vi "FaulhaberV3AsciiCommunication.vi"(8 "error in (no error)":errorcluster, 10 "Befehl":string="Statusword?", 11 "VISA resource name":refnum<visa-resource-name>="COM10") -> (0 "error out":errorcluster={"status"=FALSE, "code"=1073676293, "source"="VISA Read in FaulhaberCommunication.vi->Faulhaber_Standalone.vi"}, 1 "returnValue":i32 format="%.0x", 2 "return":string="5000\r\n", 3 "VISA resource name out":refnum<visa-resource-name>="COM10")   [LabVIEW 2011]
uses:
  FaulaberType.ctl
panel:
  out "type":T1=enum."R"
  in  "Knoten":u8=1
  out "Befehl 2":T2(ring)
  out "Value":i32 format="%.0x"
  out "Index":u32 format="%04x"
  # "2025 new binary interface"
  # "Modes of operation=1\nControlword=0xF\nControlword?\nStatusword?\nTarget position=12345\nControlword=0xF\nControlword=0xF\nPosition actual value?"
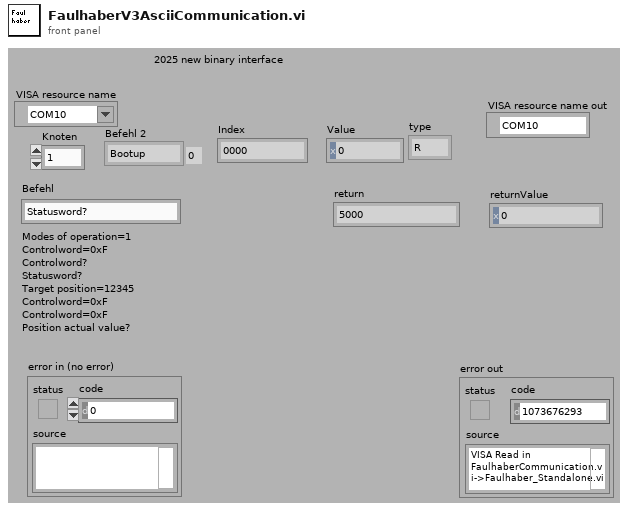
[diagram p1: front panel]
types:
  T1 = typedef "FaulaberType.ctl" = enum8{"unknown", "none", "S8", "S16", "S32", "U8", "U16", "U32", "R", "string"}
  T2 = enum8{"Bootup", "SDORead", "SDOWrite", "SDOErrror", "Controlword", "Statusword", "TraceLog", "Emcy", "SDOBlockReadInit", "SDOBlockReadUpload", "SDOBlockReadEnd", "SDOBlockWriteInit", "SDOBlockWriteDownload", "SDOBlockWriteEnd"}
  T3 = typedef "FaulhaberAccess.ctl" = enum16{"unknown", "ro", "rw", "wo", "const"}
  T4 = cluster{"ID":u32, "Name":string, "type":T1, "rw":T3, "lowLimit":string, "highLimit":string, "Default":string, "Kommentart":string}[]
  T5 = cluster{"ID":u32, "Name":string, "type":T1, "rw":T3, "lowLimit":string, "highLimit":string, "Default":string, "Kommentart":string}
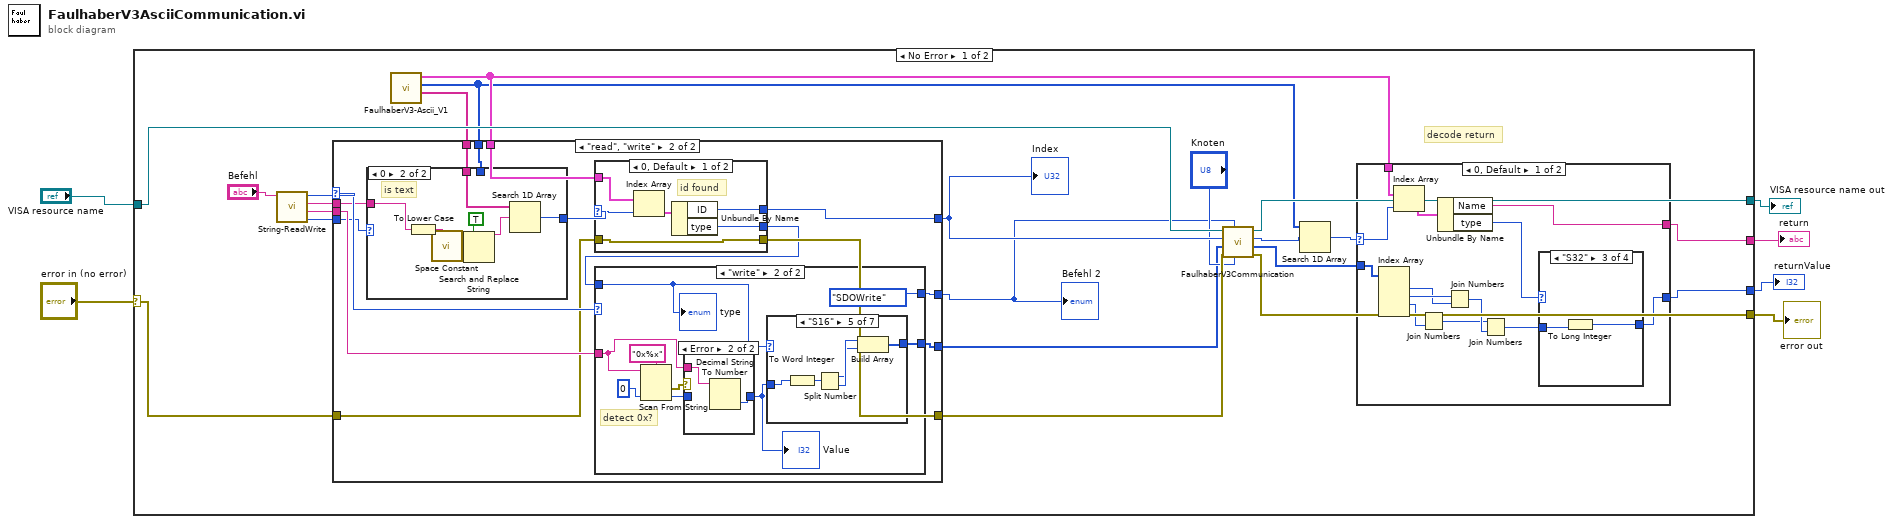
[diagram p0: block diagram]
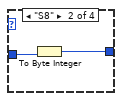
[diagram p3: hidden frame]
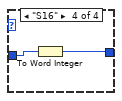
[diagram p4: hidden frame]
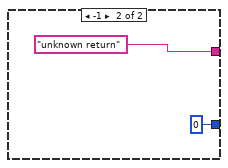
[diagram p5: hidden frame]
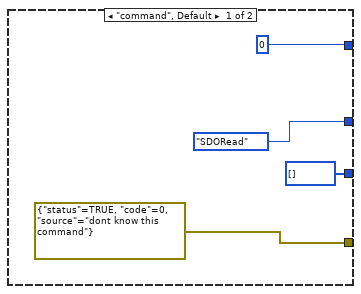
[diagram p6: hidden frame]
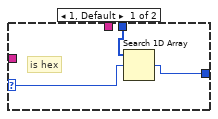
[diagram p7: hidden frame]
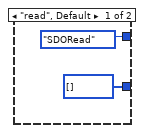
[diagram p8: hidden frame]
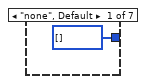
[diagram p10: hidden frame]
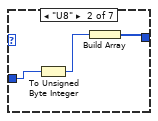
[diagram p11: hidden frame]
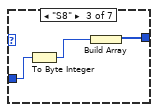
[diagram p12: hidden frame]
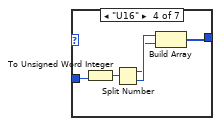
[diagram p13: hidden frame]
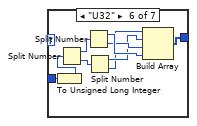
[diagram p14: hidden frame]
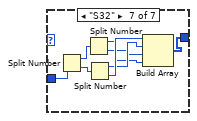
[diagram p15: hidden frame]
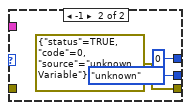
[diagram p16: hidden frame]
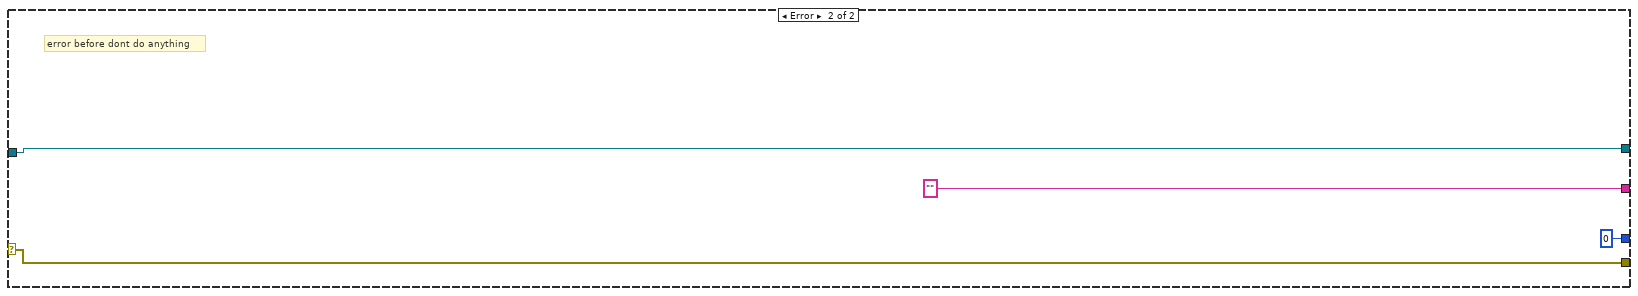
[diagram p17: hidden frame]
diagram:
  n1 = case shown="No Error" "error in (no error)" {
    selector: "error in (no error)" -> [w19 w139]
    tunnel: "VISA resource name" -> [w28 w140]
    tunnel: [w27 w140] -> w5
    tunnel: [w26 w139] -> w4
    tunnel: [w10 u32 0] -> w1
    tunnel: [w11 "" ("name")] -> w2
    frame No Error {
      # "decode return"
      n2 = call "String-ReadWrite.vi"("Befehl"="Befehl") -> ("output 1"=w9:u32, "Argument"=w22:string, "Befehl,Variable"=w23:string, "Enum"=w24:enum16{"command", "read", "write"})  [unwired: 7 in]
      n3 = call "FaulhaberV3-Ascii_V1.vi"() -> ("searchnames"=w21:string[], "ID"=w8:u32[], "Faulhaber Objects"=w13:T4)  [unwired: 9 in]
      n4 = case shown="\"read\", \"write\"" w24 {
        selector: w24 -> [_ w65]
        tunnel: w23 -> [_ w60]
        tunnel: w22 -> [_ w63]
        tunnel: w21 -> [_ w69]
        tunnel: w13 -> [_ w67]
        tunnel: [u32 0 ("ID") w66] -> w18
        tunnel: [T2."SDORead" ("Befehl 2") w64] -> w16
        tunnel: [errorcluster {"status"=TRUE, "code"=0, "source"="dont know this command"} ("error in (no error) 2") w61] -> w20
        tunnel: w19 -> [_ w62]
        tunnel: w9 -> [_ w59]
        tunnel: w8 -> [_ w58]
        tunnel: [u8[] [] w57] -> w7
        frame "command", Default {
        }
        frame "read", "write" {
          n5 = case shown="0" w59 {
            selector: w59 -> [w71 _]
            tunnel: w69 -> [_ w79]
            tunnel: [w70 w78] -> w68
            tunnel: w60 -> [_ w74]
            tunnel: w58 -> [w72 _]
            frame 1, Default {
              # "is hex"
              n6 = Search 1D Array(1D array=w72, element=w71) -> (index of element=w70:i32)  [unwired: 1 in]
            }
            frame 0 {
              # "is text"
              n7 = To Lower Case(string=w74) -> (all lower case string=w75:string)
              n8 = call <vilib>:"Space Constant.vi"() -> ("String"=w77:string)
              n9 = Search and Replace String(replace all?=TRUE ("replace all? (F)"), input string=w75, search string=w77) -> (result string=w73:string)  [unwired: 5 in, 3 out]
              n10 = Search 1D Array(1D array=w79, element=w73) -> (index of element=w78:i32)  [unwired: 1 in]
            }
          }
          n11 = case shown="0, Default" w68 {
            selector: w68 -> [w132 _]
            tunnel: w67 -> [w133 _]
            tunnel: [w130 u32 0 ("ID")] -> w66
            tunnel: [w129 FaulaberType."unknown" ("type")] -> w56
            tunnel: w62 -> [w128 _]
            tunnel: [w128 errorcluster {"status"=TRUE, "code"=0, "source"="unknown Variable"} ("error IO")] -> w61
            frame 0, Default {
              # "id found"
              n12 = Index Array(array=w133, index=w132) -> (element=w131:T5)
              n13 = Unbundle By Name(w131) -> ("ID"=w130:u32, "type"=w129:T1)
            }
            frame -1 {
            }
          }
          n14 = case shown="\"write\"" w65 {
            tunnel: [T2."SDORead" ("Befehl 2") T2."SDOWrite" ("Befehl 2")] -> w64
            tunnel: w63 -> [_ w84]
            tunnel: [u8[] [] w87] -> w57
            tunnel: w56 -> [_ w82]
            frame "read", Default {
            }
            frame "write" {
              # "detect 0x?"
              n15 = Scan From String(format string="0x%x", input string=w84, default 1=u32 0 ("default value 1")) -> (error out=w86:errorcluster, output 1=w85:u32)  [unwired: 2 in, 2 out]
              n16 = case shown="Error" w86 {
                tunnel: w85 -> [w91 _]
                tunnel: [w91 w92] -> w83
                tunnel: w84 -> [_ w93]
                frame No Error {
                }
                frame Error {
                  n17 = Decimal String To Number(string=w93) -> (number=w92:i32)  [unwired: 2 in, 1 out]
                }
              }
              "Value" <- w83
              n18 = case shown="\"S16\"" w82 {
                tunnel: w83 -> [_ w95 w98 w101 w106 w111 w120]
                tunnel: [u8[] [] w97 w99 w102 w107 w112 w121] -> w87
                frame "none", Default {
                }
                frame "U8" {
                  n19 = To Unsigned Byte Integer(number=w95) -> (unsigned 8bit integer=w96:u8)
                  n20 = Build Array(w96) -> (w97:u8[])
                }
                frame "S8" {
                  n21 = To Byte Integer(number=w98) -> (8bit integer=w100:i8)
                  n22 = Build Array(w100) -> (w99:i8[])
                }
                frame "U16" {
                  n23 = To Unsigned Word Integer(number=w101) -> (unsigned 16bit integer=w105:u16)
                  n24 = Split Number(x=w105) -> (hi(x)=w103:u8, lo(x)=w104:u8)
                  n25 = Build Array(w104, w103) -> (w102:u8[])
                }
                frame "S16" {
                  n26 = To Word Integer(number=w106) -> (16bit integer=w110:i16)
                  n27 = Split Number(x=w110) -> (hi(x)=w108:u8, lo(x)=w109:u8)
                  n28 = Build Array(w109, w108) -> (w107:u8[])
                }
                frame "U32" {
                  n29 = To Unsigned Long Integer(number=w111) -> (unsigned 32bit integer=w113:u32)
                  n30 = Split Number(x=w113) -> (hi(x)=w115:u16, lo(x)=w114:u16)
                  n31 = Split Number(x=w115) -> (hi(x)=w119:u8, lo(x)=w118:u8)
                  n32 = Split Number(x=w114) -> (hi(x)=w117:u8, lo(x)=w116:u8)
                  n33 = Build Array(w116, w117, w118, w119) -> (w112:u8[])
                }
                frame "S32" {
                  n34 = Split Number(x=w120) -> (hi(x)=w126:u16, lo(x)=w127:u16)
                  n35 = Split Number(x=w126) -> (hi(x)=w122:u8, lo(x)=w123:u8)
                  n36 = Split Number(x=w127) -> (hi(x)=w124:u8, lo(x)=w125:u8)
                  n37 = Build Array(w125, w124, w123, w122) -> (w121:u8[])
                }
              }
              "type" <- w82
            }
          }
        }
      }
      "Index" <- w18
      "Befehl 2" <- w16
      n38 = call "FaulhaberV3Communication.vi"("Knoten"="Knoten", "Befehl"=w16, "error in (no error)"=w20, "SendValue"=w7, "SendObject"=w18, "VISA resource name"=w28) -> ("error out"=w26:errorcluster, "Return Value"=w12:u8[], "RecieveObject"=w15:u32, "VISA resource name out"=w27:refnum<visa-resource-name>)  [unwired: 2 in]
      n39 = Search 1D Array(1D array=w8, element=w15) -> (index of element=w14:i32)  [unwired: 1 in]
      n40 = case shown="0, Default" w14 {
        selector: w14 -> [w41 _]
        tunnel: w13 -> [w42 _]
        tunnel: w12 -> [w34 _]
        tunnel: [w39 "unknown return" ("Name")] -> w11
        tunnel: [w29 u32 0] -> w10
        frame 0, Default {
          n41 = Index Array(array=w34) -> (element #1=w35:u8, element #2=w36:u8, element #3=w33:u8, element #4=w32:u8)  [unwired: 4 in]
          n42 = Index Array(array=w42, index=w41) -> (element=w40:T5)
          n43 = Join Numbers(hi=w32, lo=w33) -> ((hi.lo)=w37:u16)
          n44 = Unbundle By Name(w40) -> ("Name"=w39:string, "type"=w31:T1)
          n45 = Join Numbers(hi=w36, lo=w35) -> ((hi.lo)=w38:u16)
          n46 = Join Numbers(hi=w37, lo=w38) -> ((hi.lo)=w30:u32)
          n47 = case shown="\"S32\"" w31 {
            tunnel: w30 -> [w43 w45 w47 w49]
            tunnel: [w43 w44 w46 w48] -> w29
            frame "unknown", Default {
            }
            frame "S8" {
              n48 = To Byte Integer(number=w45) -> (8bit integer=w44:i8)
            }
            frame "S32" {
              n49 = To Long Integer(number=w47) -> (32bit integer=w46:i32)
            }
            frame "S16" {
              n50 = To Word Integer(number=w49) -> (16bit integer=w48:i16)
            }
          }
        }
        frame -1 {
        }
      }
    }
    frame Error {
      # "error before dont do anything"
    }
  }
  "VISA resource name out" <- w5
  "error out" <- w4
  "returnValue" <- w1
  "return" <- w2
